vi "Init MFC Gaslisten.vi"(8 "Fehler (Eingang, kein Fehler)":errorcluster, 11 "mfc Gaslisten in":string[][](array[string])) -> (0 "error out":errorcluster)   [LabVIEW 2020, in "Linearisierung v2.lvlib" / "Gasteiler.lvlib" / "HovaCAL_Interface.lvlib" / "Kommunikation.lvlib"]
uses:
  Kommunikation.lvlib
  Aktion_FGV_HovaCAL_Interface_GetData.ctl
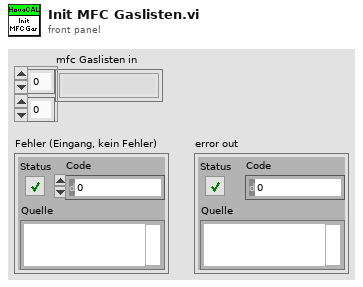
[diagram p1: front panel]
types:
  T1 = typedef "Linearisierung v2.lvlib/Gasteiler.lvlib/HovaCAL_Interface.lvlib/Kommunikation.lvlib/Aktion_FGV_HovaCAL_Interface_GetData.ctl" = enum16{"lesen", "SystemInfo", "MFC Info", "actual Values", "Limits", "first contact"}
  T2 = cluster{"System Cluster":refnum<vi>, "MFC Flow Cluster":refnum<vi>}
  T3 = cluster{"HovaCAL Limits Cluster":refnum<vi>, "HovaCAL SetPumpMode":refnum<vi>, "HovaCAL Cluster.PumpModeGeneral":refnum<vi>, "HovaCAL SetPumpMode-Cluster":refnum<vi>, "HovaCAL Flow Input Cluster":refnum<vi>, "HovaCAL Set Values Cluster":refnum<vi>[], "HovaCAL Temperature":refnum<vi>, "HovaCAL Pump Concentrations-Cluster":refnum<vi>[], "HovaCAL AutoLin MFC":refnum<vi>, "HovaCAL MFC Gase Cluster Array out":refnum<vi>[]}
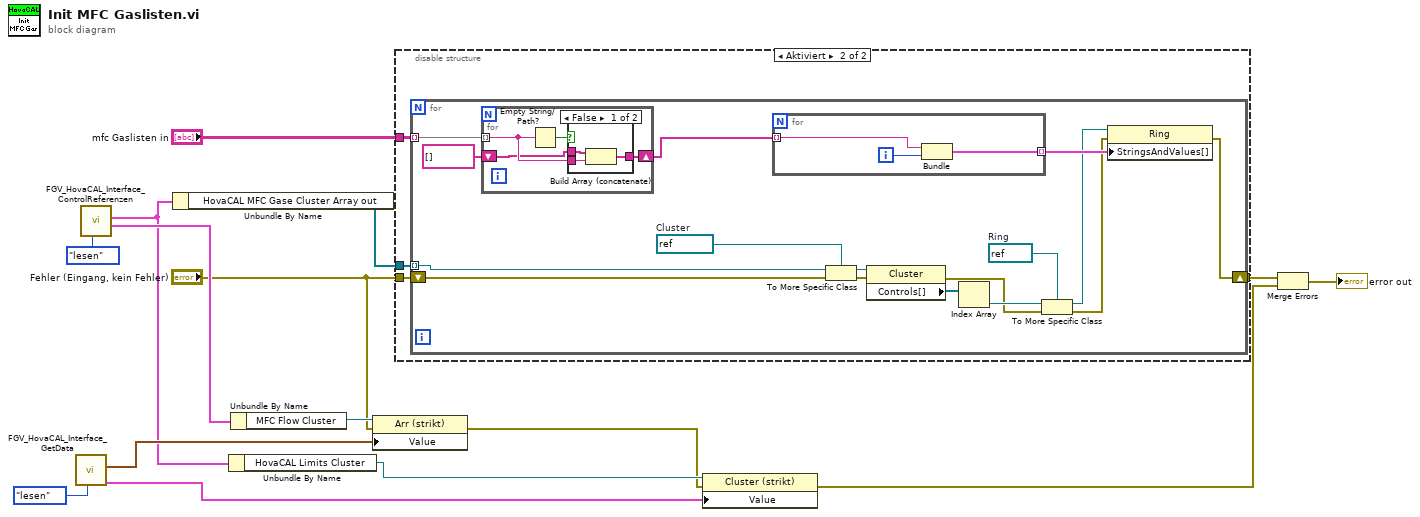
[diagram p0: block diagram]
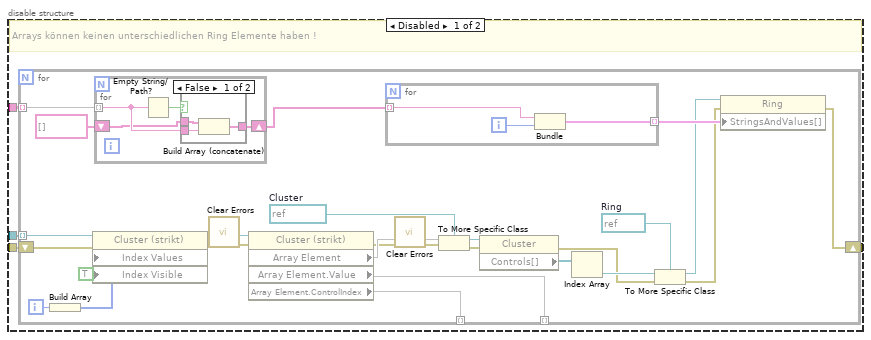
[diagram p2: hidden frame]
diagram:
  n1 = call "FGV_HovaCAL_Interface_GetData.vi"("Aktion"=Aktion_FGV_HovaCAL_Interface_GetData."lesen") -> ("Limits Cluster out"=w1:cluster{"flow":dbl[], "temp":dbl[]}, "MFC Flow Cluster out"=w7:cluster{"min flow":dbl, "max flow":dbl}[])  [unwired: 6 in, 3 out]
  n2 = call "FGV_HovaCAL_Interface_ControlReferenzen.vi"("Aktion"=enum16{"lesen", "schreiben"}."lesen") -> ("System Cluster out"=w11:T2, "Set Cluster out"=w5:T3)  [unwired: 6 in, 3 out]
  n3 = Unbundle By Name(w5) -> ("HovaCAL MFC Gase Cluster Array out"=w12:refnum<vi>[])
  n4 = Unbundle By Name(w5) -> ("HovaCAL Limits Cluster"=w4:refnum<vi>)
  n5 = Unbundle By Name(w11) -> ("MFC Flow Cluster"=w10:refnum<vi>)
  n6 = property class="Arr (strikt)"(reference=w10, error in="Fehler (Eingang, kein Fehler)", "Value"=w7) -> (error out=w3:errorcluster)  [unwired: 1 out]
  n7 = disable-structure shown="Aktiviert" {
    disable-tunnel: "mfc Gaslisten in" -> [w19 w61]
    disable-tunnel: [w18 w60] -> w13
    disable-tunnel: w12 -> [w17 w59]
    disable-tunnel: "Fehler (Eingang, kein Fehler)" -> [w16 w58]
    frame Disabled {
      # "Arrays können keinen unterschiedlichen Ring Elemente haben !"
      n8 = for {
        tunnel: w19 -> [w26] mode=indexing
        shift-right: [w45] -> w18
        shift-left: w16 -> [w30]
        tunnel: w17 -> [w34] mode=indexing
        tunnel: [w28] -> _ mode=indexing
        tunnel: [w27] -> _ mode=indexing
        i -> [w33]
        w36 = refnum<vi> refnum  # Ring
        w44 = refnum<vi> refnum  # Cluster
        n9 = Build Array(w33) -> (w32:i32[])
        n10 = property class="Cluster (strikt)"(reference=w34, error in=w30, "Index Values"=w32, "Index Visible"=TRUE ("Index sichtbar")) -> (reference out=w31:refnum<vi>, error out=w23:errorcluster)
        n11 = for {
          tunnel: w26 -> [w49] mode=indexing
          shift-right: [w48] -> w24
          shift-left: string[] [] -> [w47]
          n12 = Empty String/Path?(string/path=w49) -> (empty?=w50:bool)
          n13 = case shown="False" w50 {
            tunnel: w49 -> [w53 _]
            tunnel: [w52 w54] -> w48
            tunnel: w47 -> [w51 w54]
            frame False {
              n14 = Build Array (concatenate)(w51, w53) -> (w52:string[])
            }
            frame True {
            }
          }
        }
        n15 = call <vilib>:"Clear Errors.vi"("error in (no error)"=w23) -> ("error out"=w22:errorcluster)  [unwired: 5 in, 1 out]
        n16 = property class="Cluster (strikt)"(reference=w31, error in=w22) -> (error out=w29:errorcluster, "Array Element"=w35, "Array Element.Value"=w28, "Array Element.ControlIndex"=w27)  [unwired: 1 out]
        n17 = for {
          tunnel: w24 -> [w57] mode=indexing
          tunnel: [w55] -> w46 mode=indexing
          i -> [w56]
          n18 = Bundle("gasname"=w57, w56) -> (w55:cluster{"gasname":string, i32})  [unwired: 1 in]
        }
        n19 = call <vilib>:"Clear Errors.vi"("error in (no error)"=w29) -> ("error out"=w21:errorcluster)  [unwired: 5 in, 1 out]
        n20 = To More Specific Class(target class=w44, reference=w35, error in=w21) -> (specific class reference=w43:refnum<vi>, error out=w42:errorcluster)
        n21 = property class="Cluster"(reference=w43, error in=w42) -> (error out=w38:errorcluster, "Controls[]"=w41:refnum<vi>[])  [unwired: 1 out]
        n22 = Index Array(array=w41) -> (element=w40:refnum<vi>)  [unwired: 1 in]
        n23 = To More Specific Class(target class=w36, reference=w40, error in=w38) -> (specific class reference=w39:refnum<vi>, error out=w37:errorcluster)
        n24 = property class="Ring"(reference=w39, error in=w37, "StringsAndValues[]"=w46) -> (error out=w45:errorcluster)  [unwired: 1 out]
      }
    }
    frame Enabled {
      n25 = for {
        tunnel: w61 -> [w65] mode=indexing
        shift-right: [w76] -> w60
        shift-left: w58 -> [w66]
        tunnel: w59 -> [w62] mode=indexing
        w67 = refnum<vi> refnum  # Ring
        w75 = refnum<vi> refnum  # Cluster
        n26 = for {
          tunnel: w65 -> [w80] mode=indexing
          shift-right: [w79] -> w63
          shift-left: string[] [] -> [w78]
          n27 = Empty String/Path?(string/path=w80) -> (empty?=w81:bool)
          n28 = case shown="False" w81 {
            tunnel: w80 -> [w84 _]
            tunnel: [w83 w85] -> w79
            tunnel: w78 -> [w82 w85]
            frame False {
              n29 = Build Array (concatenate)(w82, w84) -> (w83:string[])
            }
            frame True {
            }
          }
        }
        n30 = for {
          tunnel: w63 -> [w88] mode=indexing
          tunnel: [w86] -> w77 mode=indexing
          i -> [w87]
          n31 = Bundle("gasname"=w88, w87) -> (w86:cluster{"gasname":string, i32})  [unwired: 1 in]
        }
        n32 = To More Specific Class(target class=w75, reference=w62, error in=w66) -> (specific class reference=w74:refnum<vi>, error out=w73:errorcluster)
        n33 = property class="Cluster"(reference=w74, error in=w73) -> (error out=w69:errorcluster, "Controls[]"=w72:refnum<vi>[])  [unwired: 1 out]
        n34 = Index Array(array=w72) -> (element=w71:refnum<vi>)  [unwired: 1 in]
        n35 = To More Specific Class(target class=w67, reference=w71, error in=w69) -> (specific class reference=w70:refnum<vi>, error out=w68:errorcluster)
        n36 = property class="Ring"(reference=w70, error in=w68, "StringsAndValues[]"=w77) -> (error out=w76:errorcluster)  [unwired: 1 out]
      }
    }
  }
  n37 = property class="Cluster (strikt)"(reference=w4, error in=w3, "Value"=w1) -> (error out=w2:errorcluster)  [unwired: 1 out]
  n38 = Merge Errors(w13, w2) -> (→"error out":errorcluster)
